vi "ExitCONFIG.vi"(8 "error in (no error)":errorcluster, 9 "(1)Save (0)Reverts":sgl, 10 "Address":u8, 11 "VISA resource name":refnum<visa-resource-name>) -> (0 "error out":errorcluster, 1 "Raw Response":string, 2 "(1)Saved (0)Reverted":dbl, 3 "VISA resource name out":refnum<visa-resource-name>)   [LabVIEW 2020, in "driver_flodx_rtd.lvlib"]
doc: "Exits the CONFIG state and saves/reverts your configuration changes"
uses:
  <instrlib>/RxnRover/FloDx RTD Driver/driver_flodx_rtd.lvlib
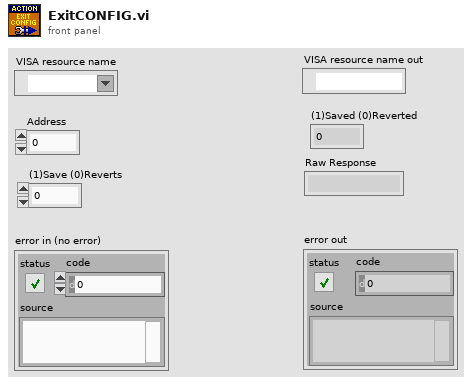
[diagram p1: front panel]
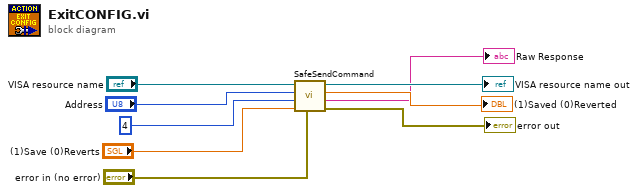
[diagram p0: block diagram]
diagram:
  n1 = call <instrlib>:"SafeSendCommand.vi"("error in"="error in (no error)", "Parameter"="(1)Save (0)Reverts", "Command #"=u8 4 ("Command"), "Address #"="Address", "VISA resource name"="VISA resource name") -> ("error out"=→"error out":errorcluster, "Raw Response"=→"Raw Response":string, "Value"=→"(1)Saved (0)Reverted":dbl, "VISA resource name out"=→"VISA resource name out":refnum<visa-resource-name>)  [unwired: 3 in]
